vi "File_setup.vi"(4 "Measurement is top level?":bool, 5 "Results file":path, 6 "Raw data file":path, 7 "setup":T1, 8 "File":T3) -> (0 "Results file output":path, 1 "Raw data file output":path, 2 "Raw data option":enum16{"Save raw data", "Raw data not saved"}(ring), 3 "File output":T2(ring))   [LabVIEW 2014]
uses:
  Controls/Save_Data.ctl
  Controls/Setup.ctl
  Controls/Post_Process.ctl
  Globals/Meas_global.vi
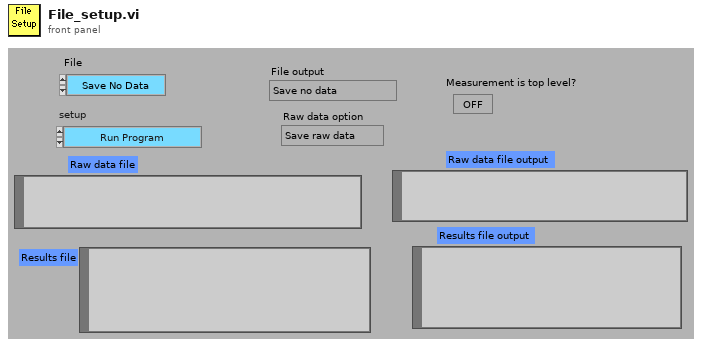
[diagram p1: front panel]
types:
  T1 = typedef "Setup.ctl" = enum16{"Run Program", "Show Setup", "Save Current Setup", "Setup Front Panel"}
  T2 = enum16{"Save no data", "Save data in new files", "Save data in existing files"}
  T3 = typedef "Save_Data.ctl" = enum16{"Save No Data", "Save Data"}
  T4 = typedef "Post_Process.ctl" = enum16{"Take New Data", "Post Process Raw Data File"}
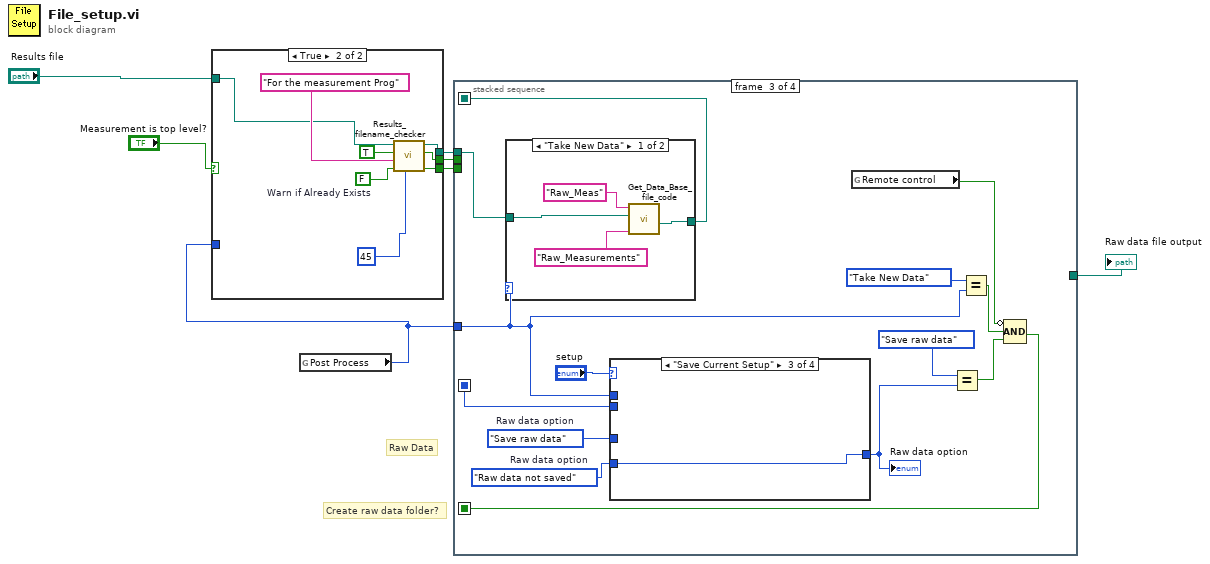
[diagram p0: block diagram]
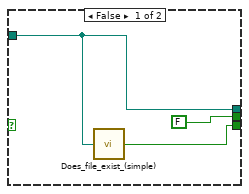
[diagram p2: hidden frame]
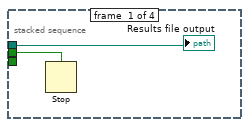
[diagram p3: hidden frame]
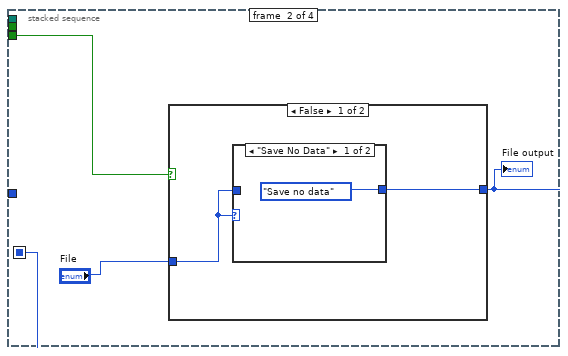
[diagram p4: hidden frame]
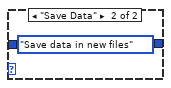
[diagram p5: hidden frame]
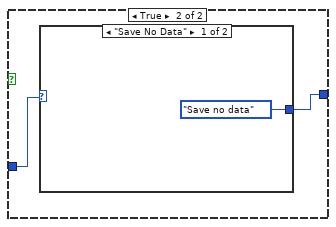
[diagram p6: hidden frame]
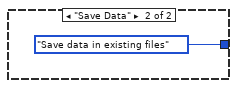
[diagram p7: hidden frame]
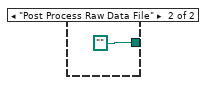
[diagram p8: hidden frame]
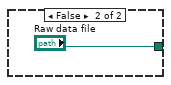
[diagram p16: hidden frame]
diagram:
  # "Create raw data folder?"
  # "Raw Data"
  n1 = global read "Meas_global.vi" "Post Process"() -> (w3:T4)
  n2 = case shown="True" "Measurement is top level?" {
    tunnel: [w10 w18] -> w7
    tunnel: [w9 w17] -> w6
    tunnel: [FALSE ("cancelled") w16] -> w4
    tunnel: w3 -> [_ _]
    tunnel: "Results file" -> [w10 w11]
    frame False {
      n3 = call "Does_file_exist_(simple).vi"("Pathname"=w10) -> ("exists?"=w9:bool)
    }
    frame True {
      w13 = FALSE  # Warn if Already Exists
      n4 = call "Results_filename_checker.vi"("Filelength"=45, "Warn if Already Exists"=w13, "Comment"="For the measurement Prog", "Show Error handler"=TRUE, "Results file"=w11) -> ("exists?"=w17:bool, "cancelled"=w16:bool, "Results file output"=w18:path)  [unwired: 1 out]
    }
  }
  n5 = stacked-sequence {
    seq-local: [_ w22 _ _] -> [_ _ w45 _]
    seq-local: [_ _ w36 _] -> [_ _ _ w69]
    seq-local: [_ _ w32 _] -> [_ _ _ w67]
    tunnel: w3 -> [_ _ w33 _]
    tunnel: w7 -> [w20 _ w35 w70]
    tunnel: w6 -> [_ w21 _ _]
    tunnel: [_ _ _ w68] -> w5
    tunnel: w4 -> [w19 _ _ _]
    frame #0 {
      n6 = Stop(stop? (T)=w19) -> ()
      "Results file output" <- w20
    }
    frame #1 {
      n7 = case shown="False" w21 {
        tunnel: "File" -> [w24 w29]
        tunnel: [w25 w28] -> w22
        frame False {
          n8 = case shown="\"Save No Data\"" w24 {
            tunnel: [T2."Save no data" ("File output") T2."Save data in new files" ("File output")] -> w25
            tunnel: w24 -> [_ _]
            frame "Save No Data" {
            }
            frame "Save Data" {
            }
          }
        }
        frame True {
          n9 = case shown="\"Save No Data\"" w29 {
            tunnel: [T2."Save no data" ("File output") T2."Save data in existing files" ("File output")] -> w28
            frame "Save No Data" {
            }
            frame "Save Data" {
            }
          }
        }
      }
      "File output" <- w22
    }
    frame #2 {
      w43 = enum16{"Save raw data", "Raw data not saved"}."Raw data not saved"  # Raw data option
      w44 = enum16{"Save raw data", "Raw data not saved"}."Save raw data"  # Raw data option
      n10 = case shown="\"Take New Data\"" w33 {
        tunnel: w35 -> [w49 _]
        tunnel: [w48 path ""] -> w32
        frame "Take New Data" {
          n11 = call "Get_Data_Base_file_code.vi"("Data Type"="Raw_Measurements", "Results Filename"=w49, "Short_Name"="Raw_Meas") -> ("Raw Data File Name"=w48:path)  [unwired: 1 in, 3 out]
        }
        frame "Post Process Raw Data File" {
        }
      }
      n12 = case shown="\"Save Current Setup\"" "setup" {
        tunnel: [w55 w64 w65 w66] -> w41
        tunnel: w43 -> [w54 w64 w65 w66]
        tunnel: w44 -> [w53 _ _ _]
        tunnel: w33 -> [w52 _ _ _]
        tunnel: w45 -> [w51 _ _ _]
        frame "Run Program" {
          n13 = case shown="\"Take New Data\"" w52 {
            tunnel: w51 -> [w59 _]
            tunnel: [w58 w63] -> w55
            tunnel: w53 -> [w57 _]
            tunnel: w54 -> [w56 w63]
            frame "Take New Data" {
              n14 = case shown="\"Save no data\"" w59 {
                tunnel: [w60 w61 w62] -> w58
                tunnel: w56 -> [w60 _ _]
                tunnel: w57 -> [_ w61 w62]
                frame "Save no data" {
                }
                frame "Save data in new files" {
                }
                frame "Save data in existing files" {
                }
              }
            }
            frame "Post Process Raw Data File" {
            }
          }
        }
        frame "Show Setup" {
        }
        frame "Save Current Setup" {
        }
        frame "Setup Front Panel" {
        }
      }
      "Raw data option" <- w41
      n15 = global read "Meas_global.vi" "Remote control"() -> (w34:bool)
      n16 = Equal?(x=enum16{"Save raw data", "Raw data not saved"}."Save raw data" ("Raw data option"), y=w41) -> (x = y?=w38:bool)
      n17 = Equal?(x=Post_Process."Take New Data" ("Post Process"), y=w33) -> (x = y?=w37:bool)
      n18 = Compound Arithmetic op=AND(invert w34, w37, w38) -> (w36:bool)
    }
    frame #3 {
      n19 = case shown="True" w69 {
        tunnel: [w71 "Raw data file"] -> w68
        tunnel: w70 -> [_ _]
        tunnel: w67 -> [w71 _]
        frame True {
        }
        frame False {
        }
      }
    }
  }
  "Raw data file output" <- w5
